vi "SupplyOutput.vi"() -> (3 "Supply Output":T1 {"Current mean" format="%0.2f"; "Voltage mean" format="%0.2f"})   [LabVIEW 2012]
uses:
  Type/SupplyOutput.ctl
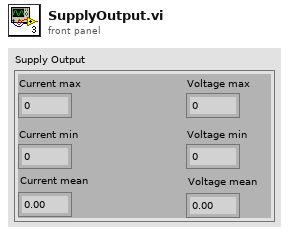
[diagram p1: front panel]
types:
  T1 = typedef "SupplyOutput.ctl" = cluster{"Current max":dbl, "Current min":dbl, "Voltage max":dbl, "Voltage min":dbl, "Voltage mean":dbl, "Current mean":dbl}
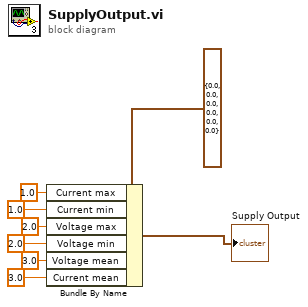
[diagram p0: block diagram]
diagram:
  n1 = Bundle By Name(cluster=T1 {"Current max"=0.0, "Current min"=0.0, "Voltage max"=0.0, "Voltage min"=0.0, "Voltage mean"=0.0, "Current mean"=0.0} ("Supply Output 2"), "Current max"=1.0, "Current min"=1.0, "Voltage max"=2.0, "Voltage min"=2.0, "Voltage mean"=3.0, "Current mean"=3.0) -> (→"Supply Output":T1)
